vi "test Verify with Regex Scrubber.vi"(8 "error in":errorcluster, 11 "Testing Approval Tests in":refnum<class "VITester Extension Tests.lvclass">) -> (0 "error out":errorcluster, 3 "Testing Approval Tests out":refnum<class "VITester Extension Tests.lvclass">)   [LabVIEW 2020, in "VITester Extension Tests.lvclass"]
uses:
  VITester Extension Tests.lvclass
  VITester Extension Tests.lvclass/VITester Extension Tests.ctl
  c85dbac9-9df1-4385-95da-0d0c429ccc49.vi
  Source/Approval Tests/Regex Scrubber/Regex Scrubber.lvclass
  Source/Approval Tests/Options/Options.lvclass
  C:/Users/SAS/Desktop/ApprovalTests.LabVIEW/Source/Approval Tests/Regex Scrubber/Regex Scrubber.lvclass
  C:/Users/SAS/Desktop/ApprovalTests.LabVIEW/Source/Approval Tests/Scrubber/Scrubber.lvclass
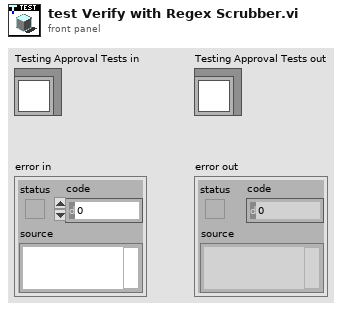
[diagram p1: front panel]
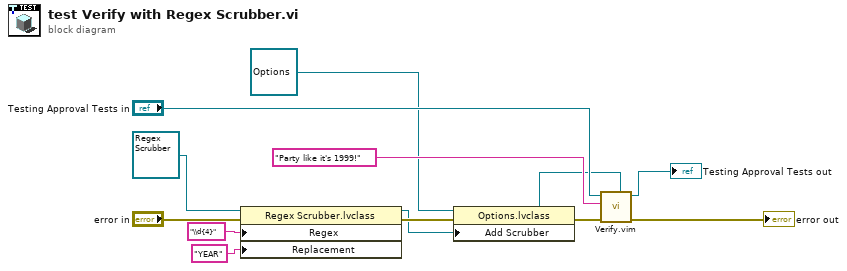
[diagram p0: block diagram]
diagram:
  n1 = property class="Regex Scrubber.lvclass"(reference=refnum<class "Regex Scrubber.lvclass"> refnum ("Approval Tests.lvlib:Regex Scrubber.lvclass"), error in="error in", "Regex"="\\d{4}", "Replacement"="YEAR") -> (reference out=w1:refnum<class "Regex Scrubber.lvclass">, error out=w12:errorcluster)
  n2 = property class="Options.lvclass"(reference=refnum<class "Options.lvclass"> refnum ("Approval Tests.lvlib:Options.lvclass"), error in=w12, "Add Scrubber"=w1) -> (reference out=w2:refnum<class "Options.lvclass">, error out=w4:errorcluster)
  n3 = call "Verify.vim"("Approval Tests.lvlib:Options.lvclass"=w2, "error in"=w4, "Test Data"="Party like it's 1999!", "TestCase"="Testing Approval Tests in") -> ("error out"=→"error out":errorcluster, "TestCase"=→"Testing Approval Tests out":refnum<class "VITester Extension Tests.lvclass">)  [unwired: 6 in]
